vi "recomendacion_uso.vi"() -> ()   [LabVIEW 2020]
panel:
  out "Waveform Chart":dbl(graph)
  out "Array 2":dbl[](array[numeric])
  out "Array":dbl[](array[numeric])
  # "for"
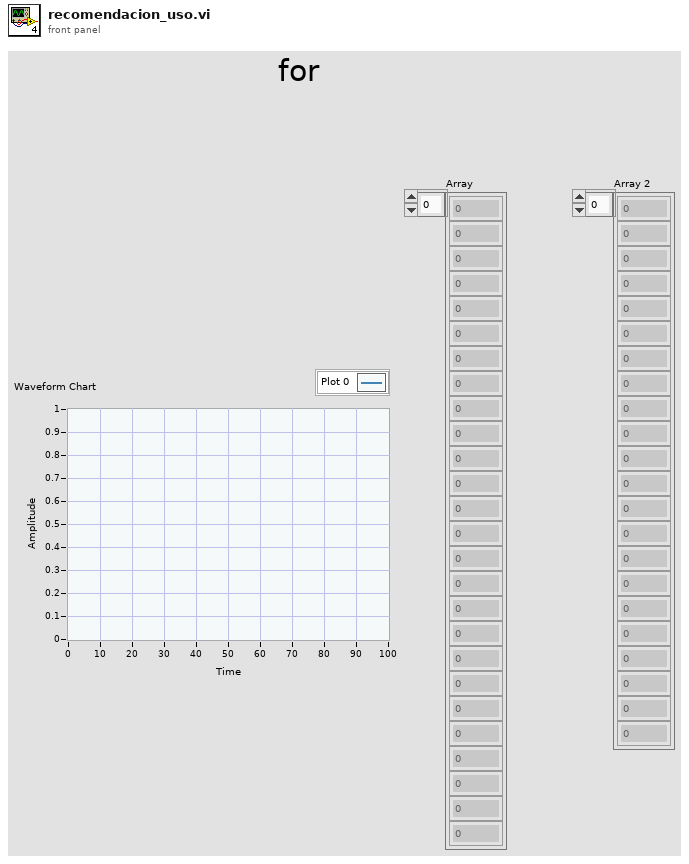
[diagram p1: front panel]
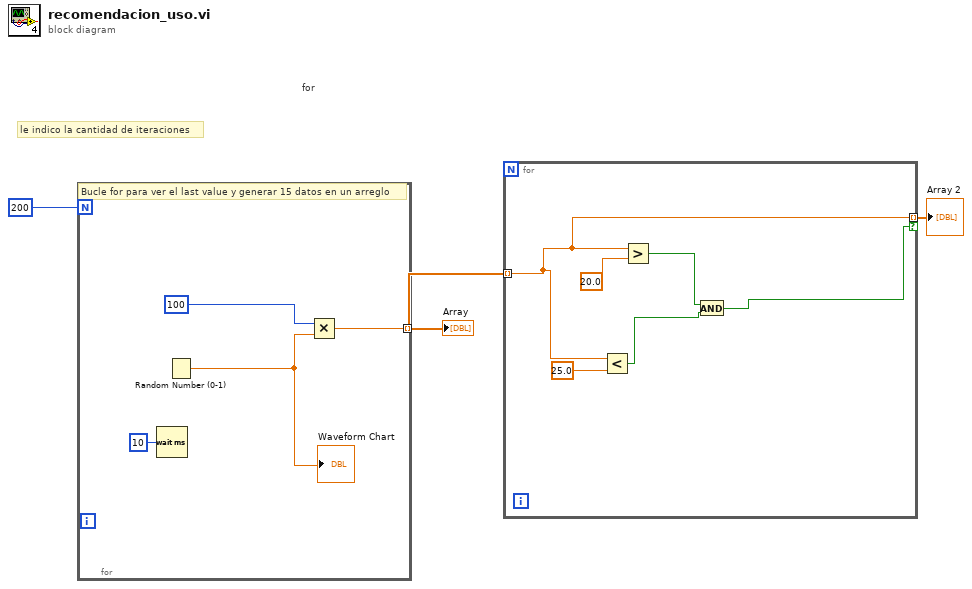
[diagram p0: block diagram]
diagram:
  # "le indico la cantidad de iteraciones"
  # "for"
  n1 = for {
    N: 200 -> [_]
    tunnel: [w6] -> w2 mode=indexing
    # "Bucle for para ver el last value y generar 15 datos en un arreglo"
    n2 = Wait (ms)(milliseconds to wait=u32 10) -> ()  [unwired: 1 out]
    n3 = Random Number (0-1)() -> (number: 0 to 1=w5:dbl)
    "Waveform Chart" <- w5
    n4 = Multiply(x=100, y=w5) -> (x*y=w6:dbl)
  }
  "Array" <- w2
  n5 = for {
    tunnel: w2 -> [w9] mode=indexing
    tunnel: [w9] -> w1 mode=indexing if=w8
    n6 = Less?(x=w9, y=25.0) -> (x < y?=w10:bool)
    n7 = Greater?(x=w9, y=20.0) -> (0:w11:bool)
    n8 = And(x=w11, y=w10) -> (x .and. y?=w8:bool)
  }
  "Array 2" <- w1
